vi "_Read.vi"(8 "error in (no error)":errorcluster, 11 "Timer in":refnum<class "Timer.lvclass">) -> (0 "error out":errorcluster, 2 "4 Data Points":dbl[](array[numeric]), 3 "Timer out":refnum<class "Timer.lvclass">)   [LabVIEW 2015, in "Timer.lvclass"]
uses:
  Timer.lvclass
  Timer.lvclass/Timer.ctl
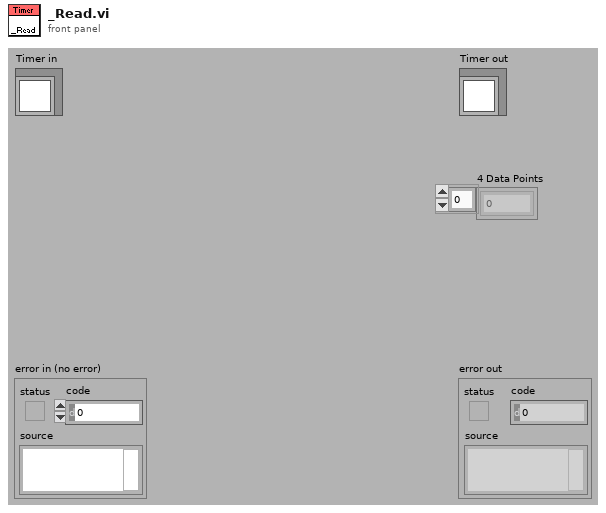
[diagram p1: front panel]
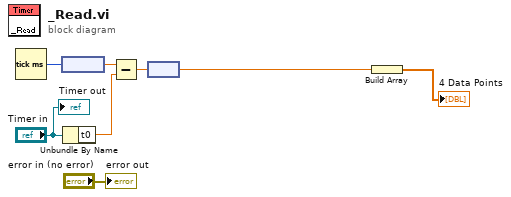
[diagram p0: block diagram]
diagram:
  n1 = Tick Count (ms)() -> (millisecond timer value=w4:u32)
  n2 = node(w4) -> (w6:dbl[unit])
  n3 = Unbundle By Name("Timer in") -> ("t0"=w7:dbl[unit])
  n4 = Subtract(x=w6, y=w7) -> (x-y=w5:dbl[unit])
  n5 = node(w5) -> (w2:dbl)
  n6 = Build Array(w2) -> (→"4 Data Points":dbl[])
  "error out" <- "error in (no error)"
  "Timer out" <- "Timer in"
